vi "check_empty_entry.vi"(4 "Problem":string, 6 "Customer Contact No.":string, 7 "Call No.":string, 9 "Engineer Name":string, 10 "Item Description":string, 11 "Customer":string) -> (3 "Boolean":bool)   [LabVIEW 2023]
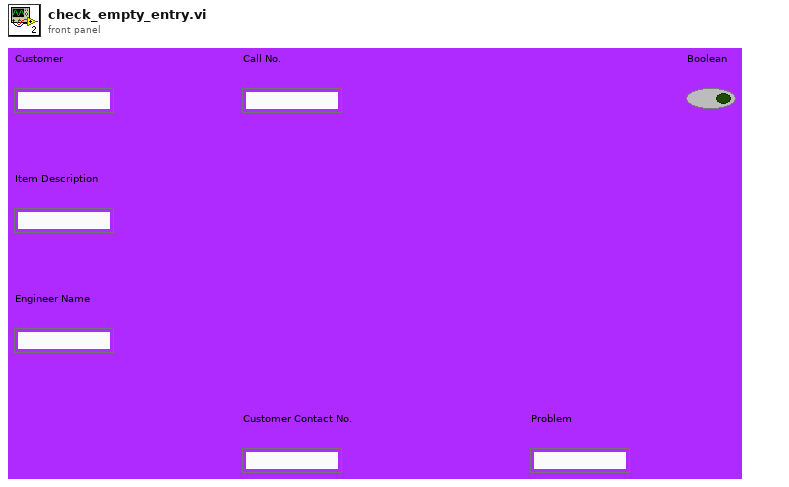
[diagram p1: front panel]
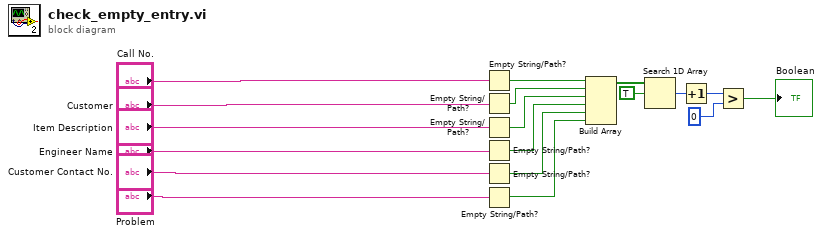
[diagram p0: block diagram]
diagram:
  n1 = Empty String/Path?(string/path="Call No.") -> (empty?=w1:bool)
  n2 = Empty String/Path?(string/path="Customer") -> (empty?=w2:bool)
  n3 = Empty String/Path?(string/path="Item Description") -> (empty?=w15:bool)
  n4 = Empty String/Path?(string/path="Engineer Name") -> (empty?=w16:bool)
  n5 = Empty String/Path?(string/path="Customer Contact No.") -> (empty?=w17:bool)
  n6 = Empty String/Path?(string/path="Problem") -> (empty?=w18:bool)
  n7 = Build Array(w1, w2, w15, w16, w17, w18) -> (w3:bool[])
  n8 = Search 1D Array(1D array=w3, element=TRUE) -> (index of element=w5:i32)  [unwired: 1 in]
  n9 = Increment(x=w5) -> (x+1=w6:i32)
  n10 = Greater?(x=w6, y=0) -> (0:→"Boolean":bool)
